vi "Lift Init.vi"   [LabVIEW 2014]
uses:
  Begin/Global Variables.vi
  Begin/Global RefNums.vi
types:
  T1 = typedef "WPI_SwitchDevRef.ctl" = cluster{"DevStatus":errorcluster, "DIO Channel":T2, "Controller":T3, "CntIndex":T4, "Normally Closed":bool}
  T2 = typedef "FPGA_DIOChannel.ctl" = enum8{"DIO 0", "DIO 1", "DIO 2", "DIO 3", "DIO 4", "DIO 5", "DIO 6", "DIO 7", "DIO 8", "DIO 9", "DIO MXP 0", "DIO MXP 1", "DIO MXP 2", "DIO MXP 3", "DIO MXP 4", "DIO MXP 5", "DIO MXP 6", "DIO MXP 7", "DIO MXP 8", "DIO MXP 9", "DIO MXP 10", "DIO MXP 11", "DIO MXP 12", "DIO MXP 13", "DIO MXP 14", "DIO MXP 15", "Invalid"}
  T3 = typedef "FPGA_TypedefDigitalModule.ctl" = enum16{"Controller 1"}
  T4 = typedef "FPGA_CounterCtrSystemIndex.ctl" = enum8{"Ctr 0", "Ctr 1", "Ctr 2", "Ctr 3", "Ctr 4", "Ctr 5", "Ctr 6", "Ctr 7", "Invalid"}
  T5 = typedef "WPI_MotorControlDeviceRef.ctl" = cluster{"DeviceStatus":errorcluster, "Type":T6, "PWM":cluster{"Controller":T3, "PWM Channel":T7, "DeadBand":T8}, "CAN":cluster{"Device Number":u8, "Control Mode":T9, "Semaphore":T10, "Max Vout":dbl, "TalonSRX Control Mode":T11}, "Invert":bool, "TransformRef":T12, "InvTransformRef":T12}
  T6 = typedef "WPI_MotorControlType.ctl" = enum16{"PWM", "CAN", "CANTalonSRX"}
  T7 = typedef "FPGA_DIOPWMChannel.ctl" = enum8{"PWM 0", "PWM 1", "PWM 2", "PWM 3", "PWM 4", "PWM 5", "PWM 6", "PWM 7", "PWM 8", "PWM 9", "PWM MXP 0", "PWM MXP 1", "PWM MXP 2", "PWM MXP 3", "PWM MXP 4", "PWM MXP 5", "PWM MXP 6", "PWM MXP 7", "PWM MXP 8", "PWM MXP 9", "Invalid"}
  T8 = typedef "WPI_PWMDeadband.ctl" = cluster{"Name":string, "maxPositivePwm":i32, "minPositivePwm":i32, "centerPwm":i32, "maxNegativePwm":i32, "minNegativePwm":i32, "angularRange":u16}
  T9 = typedef "WPI_CANJaguar_ControlMode.ctl" = enum8{"Percent VBus", "Current", "Speed", "Position", "Voltage"}
  T10 = typedef "Semaphore RefNum" = refnum<k1>
  T11 = typedef "WPI_CANTalonSRX_APIControlMode.ctl" = enum8{"Percent VBus", "Speed", "Position", "Slave", "Unchanged / Invalid"}
  T12 = typedef "WPI_PWMTransform_ConPane.ctl" = refnum<vi>
  T13 = typedef "WPI_EncoderDevRef.ctl" = cluster{"DevStatus":errorcluster, "EncoderIndex":T14, "CounterIndex":T4, "DistancePerCount":dbl, "Decoding Type":T15}
  T14 = typedef "FPGA_EncoderIdx.ctl" = enum8{"Enc 0", "Enc 1", "Enc 2", "Enc 3", "Enc 4", "Enc 5", "Enc 6", "Enc 7", "Invalid"}
  T15 = typedef "WPI_EncoderType.ctl" = enum16{"1x", "2x", "4x"}
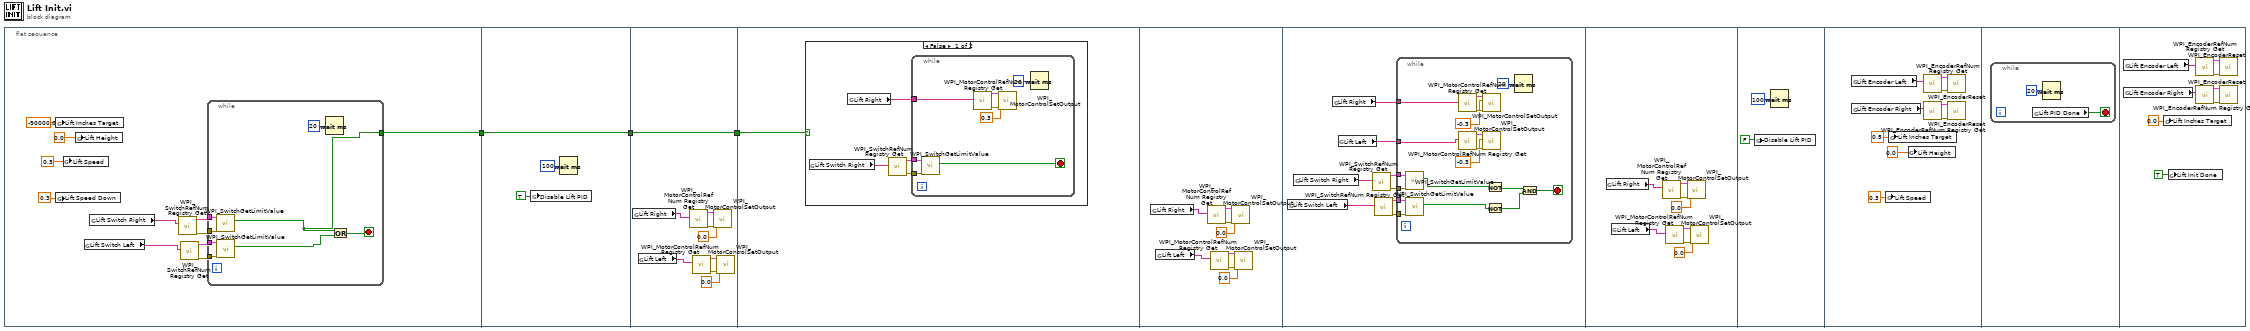
[diagram p0: block diagram]
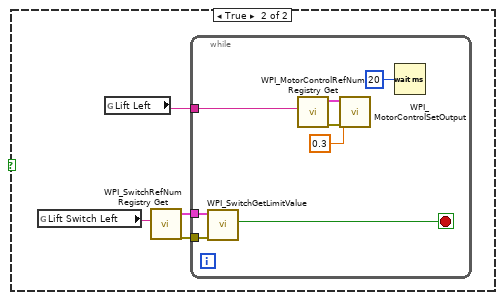
[diagram p2: hidden frame]
diagram:
  n1 = flat-sequence {
    tunnel: [w5] -> w2
    tunnel: w2 -> [w25]
    tunnel: [w25] -> w1
    tunnel: w1 -> [w34]
    tunnel: [w34] -> w3
    tunnel: w3 -> [w35]
    frame #0 {
      n2 = global write "Global Variables.vi" "Lift Inches Target"(-90000.0 ("Lift Inches Target")) -> ()
      n3 = global write "Global Variables.vi" "Lift Speed Down"(0.3 ("Lift Speed Down")) -> ()
      n4 = global write "Global Variables.vi" "Lift Speed"(0.3 ("t")) -> ()
      n5 = global write "Global Variables.vi" "Lift Height"(0.0 ("Lift Inches Target")) -> ()
      n6 = global read "Global RefNums.vi" "Lift Switch Left"() -> (w10:string)
      n7 = global read "Global RefNums.vi" "Lift Switch Right"() -> (w11:string)
      n8 = call <vilib>:"WPI_SwitchRefNum Registry Get.vi"("refnum name"=w11) -> ("error out"=w8:errorcluster, "SwitchDevRef"=w9:T1)  [unwired: 9 in]
      n9 = call <vilib>:"WPI_SwitchRefNum Registry Get.vi"("refnum name"=w10) -> ("error out"=w7:errorcluster, "SwitchDevRef"=w6:T1)  [unwired: 9 in]
      n10 = while {
        tunnel: w9 -> [w21]
        tunnel: w8 -> [w20]
        tunnel: w6 -> [w19]
        tunnel: w7 -> [w18]
        tunnel: [w15] -> w5
        stop <- w17 stop-if-true
        n11 = call <vilib>:"WPI_SwitchGetLimitValue.vi"("error in (no error)"=w20, "SwitchDevRef"=w21) -> ("Switch Pressed"=w15:bool)  [unwired: 7 in, 2 out]
        n12 = call <vilib>:"WPI_SwitchGetLimitValue.vi"("error in (no error)"=w18, "SwitchDevRef"=w19) -> ("Switch Pressed"=w16:bool)  [unwired: 7 in, 2 out]
        n13 = Wait (ms)(milliseconds to wait=u32 20) -> ()  [unwired: 1 out]
        n14 = Or(x=w15, y=w16) -> (x .or. y?=w17:bool)
      }
    }
    frame #1 {
      n15 = global write "Global Variables.vi" "Disable Lift PID"(TRUE ("Disable Lift PID")) -> ()
      n16 = Wait (ms)(milliseconds to wait=u32 100) -> ()  [unwired: 1 out]
    }
    frame #2 {
      n17 = global read "Global RefNums.vi" "Lift Right"() -> (w31:string)
      n18 = global read "Global RefNums.vi" "Lift Left"() -> (w27:string)
      n19 = call <vilib>:"WPI_MotorControlRefNum Registry Get.vi"("refnum name"=w31) -> ("error out"=w33:errorcluster, "MotorControlDevRef"=w30:T5)  [unwired: 9 in]
      n20 = call <vilib>:"WPI_MotorControlRefNum Registry Get.vi"("refnum name"=w27) -> ("error out"=w29:errorcluster, "MotorControlDevRef"=w26:T5)  [unwired: 9 in]
      n21 = call <vilib>:"WPI_MotorControlSetOutput.vi"("error in (no error)"=w33, "Output"=0.0, "MotorControlDevRef"=w30) -> ()  [unwired: 6 in, 3 out]
      n22 = call <vilib>:"WPI_MotorControlSetOutput.vi"("error in (no error)"=w29, "Output"=0.0, "MotorControlDevRef"=w26) -> ()  [unwired: 6 in, 3 out]
    }
    frame #3 {
      n23 = case shown="False" w35 {
        frame False {
          n24 = global read "Global RefNums.vi" "Lift Switch Right"() -> (w38:string)
          n25 = global read "Global RefNums.vi" "Lift Right"() -> (w39:string)
          n26 = call <vilib>:"WPI_SwitchRefNum Registry Get.vi"("refnum name"=w38) -> ("error out"=w36:errorcluster, "SwitchDevRef"=w37:T1)  [unwired: 9 in]
          n27 = while {
            tunnel: w39 -> [w44]
            tunnel: w37 -> [w43]
            tunnel: w36 -> [w42]
            stop <- w41 stop-if-true
            n28 = call <vilib>:"WPI_SwitchGetLimitValue.vi"("error in (no error)"=w42, "SwitchDevRef"=w43) -> ("Switch Pressed"=w41:bool)  [unwired: 7 in, 2 out]
            n29 = call <vilib>:"WPI_MotorControlRefNum Registry Get.vi"("refnum name"=w44) -> ("error out"=w46:errorcluster, "MotorControlDevRef"=w47:T5)  [unwired: 9 in]
            n30 = call <vilib>:"WPI_MotorControlSetOutput.vi"("error in (no error)"=w46, "Output"=0.3, "MotorControlDevRef"=w47) -> ()  [unwired: 6 in, 3 out]
            n31 = Wait (ms)(milliseconds to wait=u32 20) -> ()  [unwired: 1 out]
          }
        }
        frame True {
          n32 = global read "Global RefNums.vi" "Lift Switch Left"() -> (w49:string)
          n33 = global read "Global RefNums.vi" "Lift Left"() -> (w48:string)
          n34 = call <vilib>:"WPI_SwitchRefNum Registry Get.vi"("refnum name"=w49) -> ("error out"=w50:errorcluster, "SwitchDevRef"=w51:T1)  [unwired: 9 in]
          n35 = while {
            tunnel: w51 -> [w56]
            tunnel: w50 -> [w55]
            tunnel: w48 -> [w54]
            stop <- w53 stop-if-true
            n36 = call <vilib>:"WPI_SwitchGetLimitValue.vi"("error in (no error)"=w55, "SwitchDevRef"=w56) -> ("Switch Pressed"=w53:bool)  [unwired: 7 in, 2 out]
            n37 = call <vilib>:"WPI_MotorControlRefNum Registry Get.vi"("refnum name"=w54) -> ("error out"=w58:errorcluster, "MotorControlDevRef"=w59:T5)  [unwired: 9 in]
            n38 = call <vilib>:"WPI_MotorControlSetOutput.vi"("error in (no error)"=w58, "Output"=0.3, "MotorControlDevRef"=w59) -> ()  [unwired: 6 in, 3 out]
            n39 = Wait (ms)(milliseconds to wait=u32 20) -> ()  [unwired: 1 out]
          }
        }
      }
    }
    frame #4 {
      n40 = global read "Global RefNums.vi" "Lift Right"() -> (w65:string)
      n41 = global read "Global RefNums.vi" "Lift Left"() -> (w61:string)
      n42 = call <vilib>:"WPI_MotorControlRefNum Registry Get.vi"("refnum name"=w65) -> ("error out"=w67:errorcluster, "MotorControlDevRef"=w64:T5)  [unwired: 9 in]
      n43 = call <vilib>:"WPI_MotorControlRefNum Registry Get.vi"("refnum name"=w61) -> ("error out"=w63:errorcluster, "MotorControlDevRef"=w60:T5)  [unwired: 9 in]
      n44 = call <vilib>:"WPI_MotorControlSetOutput.vi"("error in (no error)"=w67, "Output"=0.0, "MotorControlDevRef"=w64) -> ()  [unwired: 6 in, 3 out]
      n45 = call <vilib>:"WPI_MotorControlSetOutput.vi"("error in (no error)"=w63, "Output"=0.0, "MotorControlDevRef"=w60) -> ()  [unwired: 6 in, 3 out]
    }
    frame #5 {
      n46 = global read "Global RefNums.vi" "Lift Switch Left"() -> (w68:string)
      n47 = global read "Global RefNums.vi" "Lift Switch Right"() -> (w74:string)
      n48 = global read "Global RefNums.vi" "Lift Right"() -> (w75:string)
      n49 = global read "Global RefNums.vi" "Lift Left"() -> (w71:string)
      n50 = call <vilib>:"WPI_SwitchRefNum Registry Get.vi"("refnum name"=w74) -> ("error out"=w72:errorcluster, "SwitchDevRef"=w73:T1)  [unwired: 9 in]
      n51 = call <vilib>:"WPI_SwitchRefNum Registry Get.vi"("refnum name"=w68) -> ("error out"=w69:errorcluster, "SwitchDevRef"=w70:T1)  [unwired: 9 in]
      n52 = while {
        tunnel: w75 -> [w90]
        tunnel: w73 -> [w89]
        tunnel: w72 -> [w88]
        tunnel: w71 -> [w84]
        tunnel: w70 -> [w83]
        tunnel: w69 -> [w82]
        stop <- w81 stop-if-true
        n53 = call <vilib>:"WPI_SwitchGetLimitValue.vi"("error in (no error)"=w88, "SwitchDevRef"=w89) -> ("Switch Pressed"=w78:bool)  [unwired: 7 in, 2 out]
        n54 = call <vilib>:"WPI_SwitchGetLimitValue.vi"("error in (no error)"=w82, "SwitchDevRef"=w83) -> ("Switch Pressed"=w76:bool)  [unwired: 7 in, 2 out]
        n55 = call <vilib>:"WPI_MotorControlRefNum Registry Get.vi"("refnum name"=w90) -> ("error out"=w92:errorcluster, "MotorControlDevRef"=w93:T5)  [unwired: 9 in]
        n56 = call <vilib>:"WPI_MotorControlRefNum Registry Get.vi"("refnum name"=w84) -> ("error out"=w86:errorcluster, "MotorControlDevRef"=w80:T5)  [unwired: 9 in]
        n57 = call <vilib>:"WPI_MotorControlSetOutput.vi"("error in (no error)"=w92, "Output"=-0.3 ("right side  2"), "MotorControlDevRef"=w93) -> ()  [unwired: 6 in, 3 out]
        n58 = call <vilib>:"WPI_MotorControlSetOutput.vi"("error in (no error)"=w86, "Output"=-0.3 ("right side  2"), "MotorControlDevRef"=w80) -> ()  [unwired: 6 in, 3 out]
        n59 = Not(x=w78) -> (.not. x?=w79:bool)
        n60 = Not(x=w76) -> (.not. x?=w77:bool)
        n61 = Wait (ms)(milliseconds to wait=u32 20) -> ()  [unwired: 1 out]
        n62 = And(x=w79, y=w77) -> (x .and. y?=w81:bool)
      }
    }
    frame #6 {
      n63 = global read "Global RefNums.vi" "Lift Right"() -> (w99:string)
      n64 = global read "Global RefNums.vi" "Lift Left"() -> (w95:string)
      n65 = call <vilib>:"WPI_MotorControlRefNum Registry Get.vi"("refnum name"=w99) -> ("error out"=w101:errorcluster, "MotorControlDevRef"=w98:T5)  [unwired: 9 in]
      n66 = call <vilib>:"WPI_MotorControlRefNum Registry Get.vi"("refnum name"=w95) -> ("error out"=w97:errorcluster, "MotorControlDevRef"=w94:T5)  [unwired: 9 in]
      n67 = call <vilib>:"WPI_MotorControlSetOutput.vi"("error in (no error)"=w101, "Output"=0.0, "MotorControlDevRef"=w98) -> ()  [unwired: 6 in, 3 out]
      n68 = call <vilib>:"WPI_MotorControlSetOutput.vi"("error in (no error)"=w97, "Output"=0.0, "MotorControlDevRef"=w94) -> ()  [unwired: 6 in, 3 out]
    }
    frame #7 {
      n69 = global write "Global Variables.vi" "Disable Lift PID"(FALSE ("Disable Lift PID")) -> ()
      n70 = Wait (ms)(milliseconds to wait=u32 100) -> ()  [unwired: 1 out]
    }
    frame #8 {
      n71 = global read "Global RefNums.vi" "Lift Encoder Left"() -> (w109:string)
      n72 = global read "Global RefNums.vi" "Lift Encoder Right"() -> (w108:string)
      n73 = global write "Global Variables.vi" "Lift Speed"(0.3 ("Lift Speed")) -> ()
      n74 = global write "Global Variables.vi" "Lift Inches Target"(0.5 ("Lift Inches Target")) -> ()
      n75 = global write "Global Variables.vi" "Lift Height"(0.0 ("Lift Inches Target")) -> ()
      n76 = call <vilib>:"WPI_EncoderRefNum Registry Get.vi"("refnum name"=w109) -> ("error out"=w112:errorcluster, "EncoderDevRef"=w107:T13)  [unwired: 9 in]
      n77 = call <vilib>:"WPI_EncoderRefNum Registry Get.vi"("refnum name"=w108) -> ("error out"=w110:errorcluster, "EncoderDevRef"=w111:T13)  [unwired: 9 in]
      n78 = call <vilib>:"WPI_EncoderReset.vi"("error in (no error)"=w112, "EncoderDevRef"=w107) -> ()  [unwired: 8 in, 2 out]
      n79 = call <vilib>:"WPI_EncoderReset.vi"("error in (no error)"=w110, "EncoderDevRef"=w111) -> ()  [unwired: 8 in, 2 out]
    }
    frame #9 {
      n80 = while {
        stop <- w113 stop-if-true
        n81 = global read "Global Variables.vi" "Lift PID Done"() -> (w113:bool)
        n82 = Wait (ms)(milliseconds to wait=u32 20) -> ()  [unwired: 1 out]
      }
    }
    frame #10 {
      n83 = global read "Global RefNums.vi" "Lift Encoder Left"() -> (w121:string)
      n84 = global read "Global RefNums.vi" "Lift Encoder Right"() -> (w122:string)
      n85 = global write "Global Variables.vi" "Lift Inches Target"(0.0 ("Lift Inches Target")) -> ()
      n86 = global write "Global Variables.vi" "Lift Init Done"(TRUE ("Lift Init Done")) -> ()
      n87 = call <vilib>:"WPI_EncoderRefNum Registry Get.vi"("refnum name"=w121) -> ("error out"=w118:errorcluster, "EncoderDevRef"=w117:T13)  [unwired: 9 in]
      n88 = call <vilib>:"WPI_EncoderRefNum Registry Get.vi"("refnum name"=w122) -> ("error out"=w120:errorcluster, "EncoderDevRef"=w119:T13)  [unwired: 9 in]
      n89 = call <vilib>:"WPI_EncoderReset.vi"("error in (no error)"=w118, "EncoderDevRef"=w117) -> ()  [unwired: 8 in, 2 out]
      n90 = call <vilib>:"WPI_EncoderReset.vi"("error in (no error)"=w120, "EncoderDevRef"=w119) -> ()  [unwired: 8 in, 2 out]
    }
  }
